vi "Special Schemes.vi"() -> (2 "Special Schemes":string[][](array[string])=[["ftp", "21"], ["file", "0"], ["http", "80"], ["https", "443"], ["ws", "80"], ["wss", "433"]])   [LabVIEW 2020, in "Stream.lvlib" / "URLPattern.lvclass"]
uses:
  URLPattern.lvclass
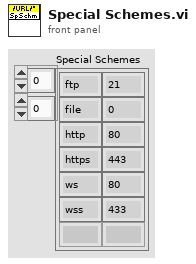
[diagram p1: front panel]
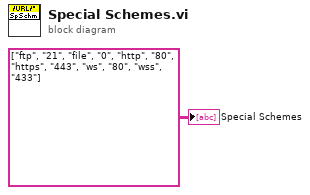
[diagram p0: block diagram]
diagram:
  "Special Schemes" <- string[][] [["ftp", "21"], ["file", "0"], ["http", "80"], ["https", "443"], ["ws", "80"], ["wss", "433"]]
